vi "x-y-z검사.vi"() -> ()   [LabVIEW 2021]
uses:
  <vilib>/DAQmx/read.llb/DAQmx Read (Analog 1D Wfm NChan NSamp).vi
  <vilib>/DAQmx/create/channels.llb/DAQmx Create Channel (AI-Voltage-Basic).vi
  <vilib>/DAQmx/configure/timing.llb/DAQmx Timing (Sample Clock).vi
  <vilib>/DAQmx/miscellaneous.llb/DAQmx Fill In Error Info.vi
  <vilib>/DAQmx/read.llb/DAQmx Read (Analog DBL 1Chan 1Samp).vi
  <vilib>/DAQmx/read.llb/DAQmx Read (Analog Wfm 1Chan NSamp).vi
panel:
  out "원소":waveform(dbl)(graph)
  out "data":waveform(dbl)[](array[waveform]) caption="데이터"
  out "x-y":u32
  in  "정지 2":bool
  out "웨이브폼 차트 3":waveform(dbl)[](graph)
  out "웨이브폼 차트 2":waveform(dbl)(graph)
  out "웨이브폼 차트":dbl(graph)
  in  "정지":bool
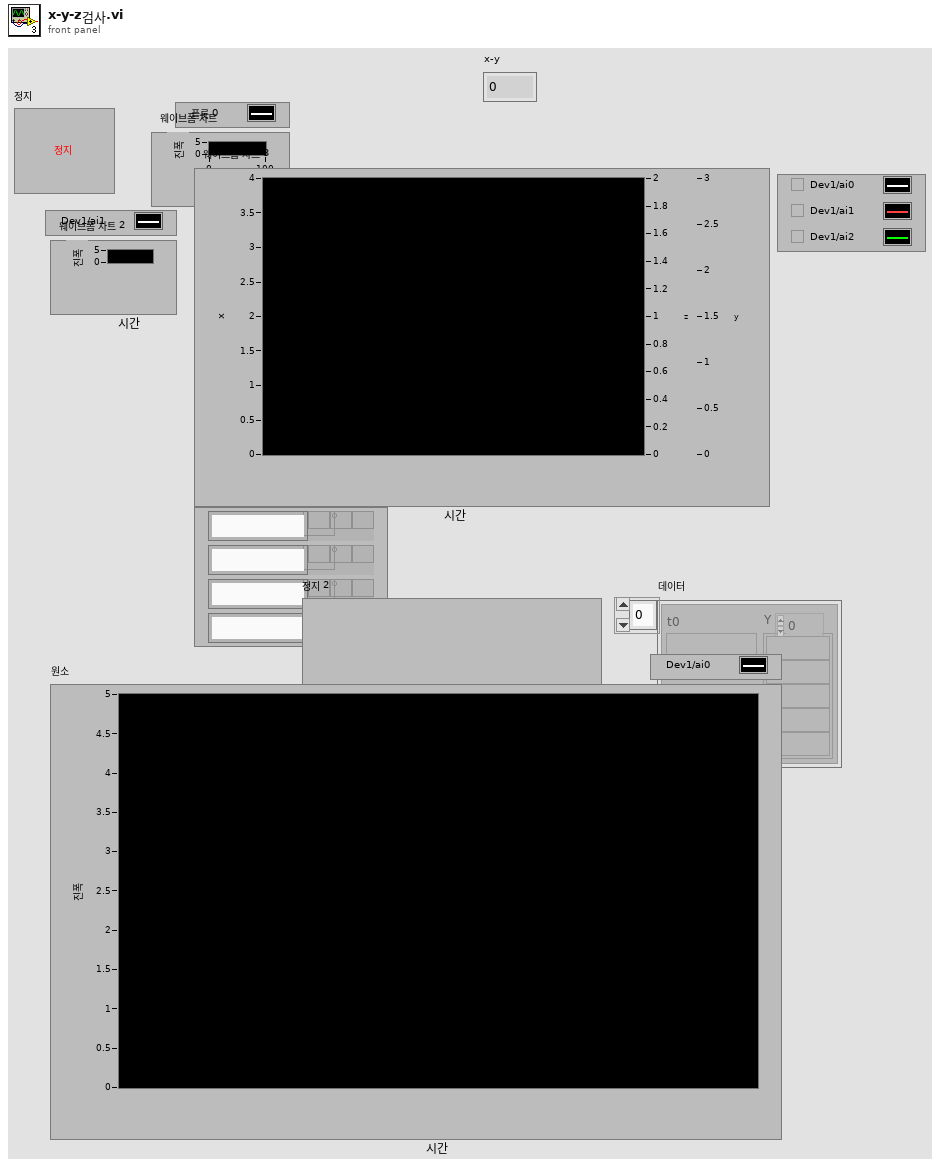
[diagram p1: front panel]
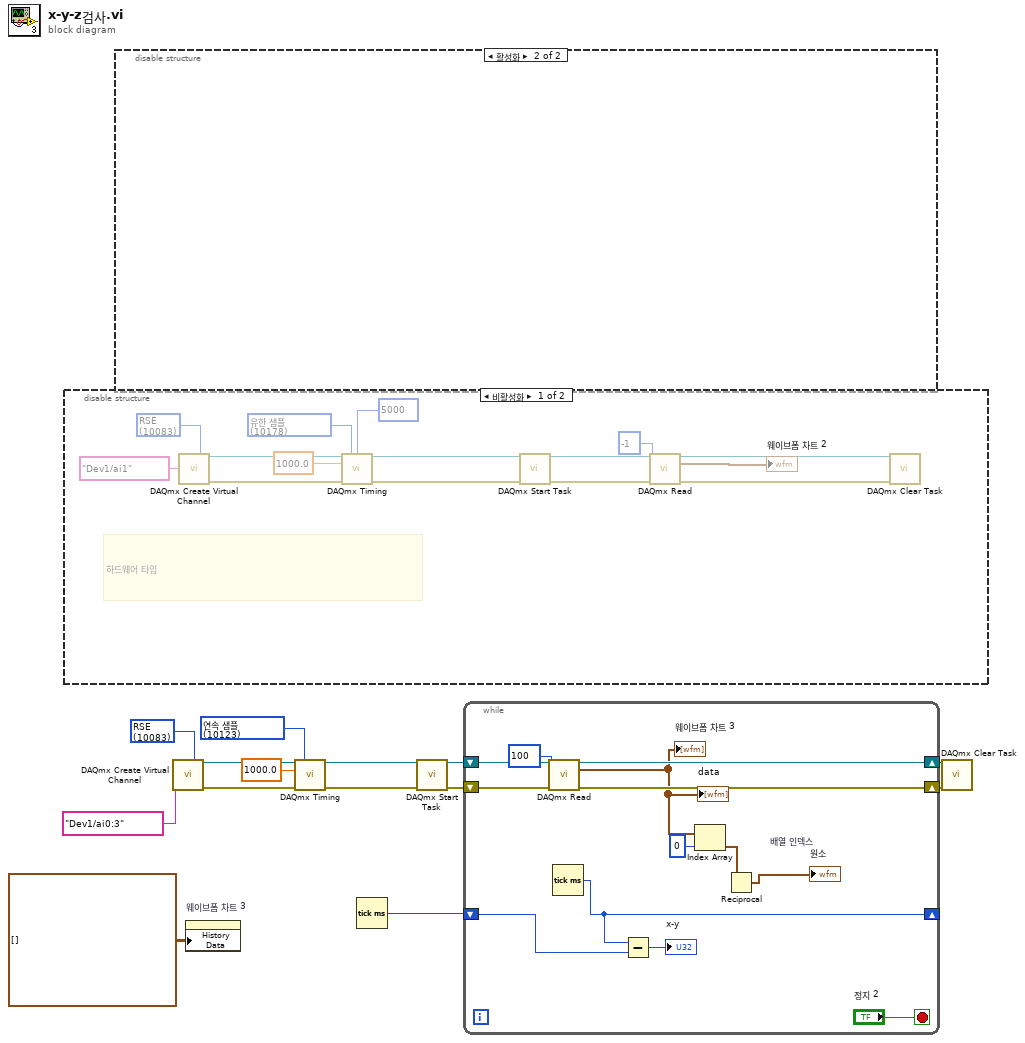
[diagram p0: block diagram]
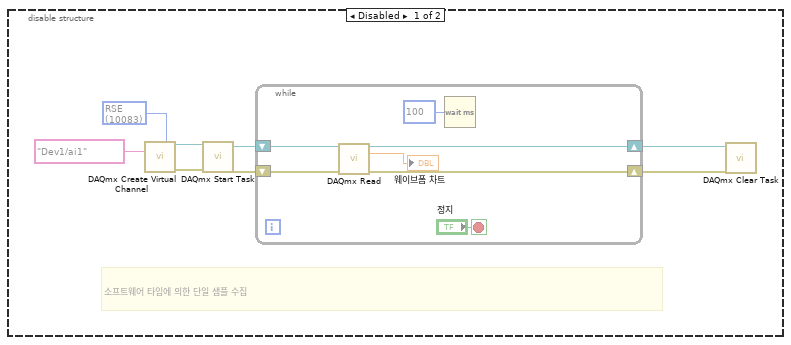
[diagram p3: hidden frame]
diagram:
  w3 = 10123 items=["유한 샘플"=10178, "연속 샘플"=10123, "하드웨어 타이밍에 의한 단일 포인트"=12522] ("sample mode")
  w5 = 10083 items=["기본"=-1, "RSE"=10083, "NRSE"=10078, "차동"=10106, "유사 차동"=12529] ("input terminal configuration")
  n1 = disable-structure shown="비활성화" {
    frame Disabled {
      w21 = 10178 items=["유한 샘플"=10178, "연속 샘플"=10123, "하드웨어 타이밍에 의한 단일 포인트"=12522] ("sample mode")
      w22 = 10083 items=["기본"=-1, "RSE"=10083, "NRSE"=10078, "차동"=10106, "유사 차동"=12529] ("input terminal configuration")
      # "하드웨어 타임"
      n2 = call-poly <vilib>:"DAQmx Create Virtual Channel.vi"("input terminal configuration"=w22, "physical channels"=tag "Dev1/ai1") -> ("task out"=w29:refnum<k21>, "error out"=w28:errorcluster)  [unwired: 12 in]
      n3 = call-poly <vilib>:"DAQmx Timing.vi"("task/channels in"=w29, "sample mode"=w21, "samples per channel"=5000, "rate"=1000.0, "error in"=w28) -> ("task out"=w27:refnum<k21>, "error out"=w26:errorcluster)  [unwired: 9 in]
      n4 = call <vilib>:"DAQmx Start Task.vi"("task/channels in"=w27, "error in"=w26) -> ("task out"=w25:refnum<k21>, "error out"=w24:errorcluster)  [unwired: 12 in]
      n5 = call-poly <vilib>:"DAQmx Read.vi"("task/channels in"=w25, "number of samples per channel"=-1, "error in"=w24) -> ("task out"=w16:refnum<k21>, "data"=→"웨이브폼 차트 2":waveform(dbl), "error out"=w15:errorcluster)  [unwired: 10 in]
      n6 = call <vilib>:"DAQmx Clear Task.vi"("task in"=w16, "error in"=w15) -> ()  [unwired: 13 in, 1 out]
    }
    frame Enabled {
    }
  }
  n7 = disable-structure shown="활성화" {
    frame Disabled {
      w30 = 10083 items=["기본"=-1, "RSE"=10083, "NRSE"=10078, "차동"=10106, "유사 차동"=12529] ("input terminal configuration")
      # "소프트웨어 타임에 의한 단일 샘플 수집"
      n8 = call-poly <vilib>:"DAQmx Create Virtual Channel.vi"("input terminal configuration"=w30, "physical channels"=tag "Dev1/ai1") -> ("task out"=w37:refnum<k21>, "error out"=w36:errorcluster)  [unwired: 12 in]
      n9 = call <vilib>:"DAQmx Start Task.vi"("task/channels in"=w37, "error in"=w36) -> ("task out"=w35:refnum<k21>, "error out"=w34:errorcluster)  [unwired: 12 in]
      n10 = while {
        shift-right: [w42] -> w33
        shift-left: w35 -> [w44]
        shift-right: [w41] -> w32
        shift-left: w34 -> [w43]
        stop <- "정지" stop-if-true
        n11 = call-poly <vilib>:"DAQmx Read.vi"("task/channels in"=w44, "error in"=w43) -> ("task out"=w42:refnum<k21>, "data"=→"웨이브폼 차트":dbl, "error out"=w41:errorcluster)  [unwired: 11 in]
        n12 = Wait (ms)(milliseconds to wait=u32 100 ("대기 시간 (ms)")) -> ()  [unwired: 1 out]
      }
      n13 = call <vilib>:"DAQmx Clear Task.vi"("task in"=w33, "error in"=w32) -> ()  [unwired: 13 in, 1 out]
    }
    frame Enabled {
    }
  }
  n14 = call-poly <vilib>:"DAQmx Create Virtual Channel.vi"("input terminal configuration"=w5, "physical channels"=tag "Dev1/ai0:3") -> ("task out"=w14:refnum<k21>, "error out"=w13:errorcluster)  [unwired: 12 in]
  n15 = property on="웨이브폼 차트 3" class="WFChart (엄격한)"("History Data"=waveform(dbl)[][] [] ("히스토리 데이터")) -> ()  [unwired: 2 in, 2 out]
  n16 = call-poly <vilib>:"DAQmx Timing.vi"("task/channels in"=w14, "sample mode"=w3, "rate"=1000.0, "error in"=w13) -> ("task out"=w12:refnum<k21>, "error out"=w11:errorcluster)  [unwired: 10 in]
  n17 = Tick Count (ms)() -> (millisecond timer value=w2:u32)
  n18 = call <vilib>:"DAQmx Start Task.vi"("task/channels in"=w12, "error in"=w11) -> ("task out"=w10:refnum<k21>, "error out"=w9:errorcluster)  [unwired: 12 in]
  n19 = while {
    shift-right: [w55] -> w8
    shift-left: w10 -> [w57]
    shift-right: [w54] -> w7
    shift-left: w9 -> [w56]
    shift-right: [w52] -> _
    shift-left: w2 -> [w51]
    stop <- "정지 2" stop-if-true
    n20 = call-poly <vilib>:"DAQmx Read.vi"("task/channels in"=w57, "number of samples per channel"=100, "error in"=w56) -> ("task out"=w55:refnum<k21>, "data"=w48:waveform(dbl)[], "error out"=w54:errorcluster)  [unwired: 10 in]
    "웨이브폼 차트 3" <- w48
    "data" <- w48
    n21 = Tick Count (ms)() -> (millisecond timer value=w52:u32)
    n22 = Subtract(x=w52, y=w51) -> (x-y=→"x-y":u32)
    n23 = Index Array "배열 인덱스"(array=w48, index=0 ("인덱스")) -> (element=w46:waveform(dbl))
    n24 = Reciprocal(x=w46) -> (1/x=→"원소":waveform(dbl))
  }
  n25 = call <vilib>:"DAQmx Clear Task.vi"("task in"=w8, "error in"=w7) -> ()  [unwired: 13 in, 1 out]
